vi "Test Deserialize Variant Attributes.vi"(8 "error in (no error)":errorcluster) -> (0 "error out":errorcluster)   [LabVIEW 2015]
uses:
  src/Deserializer/JSON Deserializer/JSON Deserializer.lvclass
  <vilib>/addons/_JKI Toolkits/Caraya/classes/Test/Test.lvclass
  <vilib>/addons/_JKI Toolkits/Caraya/classes/Assert/Assert.lvclass
  <vilib>/Utility/Data Type/NI_Data Type.lvlib
panel:
  out "element":variant
  out "value 2":variant
  out "data 2":string
  out "value":variant
  in  "Google reverse-geocode results":string="{\n   \"results\" : [\n      {\n         \"address_components\" : [\n            {\n               \"long_name\" : \"The White House\",\n               \"short_name\" : \"The White House\",\n               \"types\" : [ \"premise\" ]\n            },\n            {\n               \"long_name\" : \"1600\",\n               \"short_name\" : \"1600\",\n               \"types\" : [ \"street_number\" ]\n            },\n            {\n               \"long_name\" : \"Pennsylvania Avenue Northwest\",\n               \"short_name\" : \"Pennsylvania Ave NW\",\n               \"types\" : [ \"route\" ]\n            },\n            {\n               \"long_name\" : \"Northwest Washington\",\n               \"short_name\" : \"Northwest Washington\",\n               \"types\" : [ \"neighborhood\", \"political\" ]\n            },\n            {\n               \"long_name\" : \"Washington\",\n               \"short_name\" : \"Washington\",\n               \"types\" : [ \"locality\", \"political\" ]\n            },\n            {\n               \"long_name\" : \"District of Columbia\",\n               \"short_name\" : \"DC\",\n               \"types\" : [ \"administrative_area_level_1\", \"political\" ]\n            },\n            {\n               \"long_name\" : \"United States\",\n               \"short_name\" : \"US\",\n               \"types\" : [ \"country\", \"political\" ]\n            },\n            {\n               \"long_name\" : \"20500\",\n               \"short_name\" : \"20500\",\n               \"types\" : [ \"postal_code\" ]\n            }\n         ],\n         \"formatted_address\" : \"The White House, 1600 Pennsylvania Ave NW, Washington, DC 20500, USA\",\n         \"geometry\" : {\n            \"bounds\" : {\n               \"northeast\" : {\n                  \"lat\" : 38.8979044,\n                  \"lng\" : -77.0355124\n               },\n               \"southwest\" : {\n                  \"lat\" : 38.8973144,\n                  \"lng\" : -77.03795749999999\n               }\n            },\n            \"location\" : {\n               \"lat\" : 38.8976094,\n               \"lng\" : -77.0367349\n            },\n            \"location_type\" : \"ROOFTOP\",\n            \"viewport\" : {\n               \"northeast\" : {\n                  \"lat\" : 38.8989583802915,\n                  \"lng\" : -77.03538596970849\n               },\n               \"southwest\" : {\n                  \"lat\" : 38.8962604197085,\n                  \"lng\" : -77.03808393029151\n               }\n            }\n         },\n         \"place_id\" : \"ChIJGVtI4by3t4kRr51d_Qm_x58\",\n         \"types\" : [ \"premise\" ]\n      },\n      {\n         \"address_components\" : [\n            {\n               \"long_name\" : \"West Executive Avenue Northwest\",\n               \"short_name\" : \"W Executive Ave NW\",\n               \"types\" : [ \"route\" ]\n            },\n            {\n               \"long_name\" : \"Northwest Washington\",\n               \"short_name\" : \"Northwest Washington\",\n               \"types\" : [ \"neighborhood\", \"political\" ]\n            },\n            {\n               \"long_name\" : \"Washington\",\n               \"short_name\" : \"Washington\",\n               \"types\" : [ \"locality\", \"political\" ]\n            },\n            {\n               \"long_name\" : \"District of Columbia\",\n               \"short_name\" : \"DC\",\n               \"types\" : [ \"administrative_area_level_1\", \"political\" ]\n            },\n            {\n               \"long_name\" : \"United States\",\n               \"short_name\" : \"US\",\n               \"types\" : [ \"country\", \"political\" ]\n            },\n            {\n               \"long_name\" : \"20500\",\n               \"short_name\" : \"20500\",\n               \"types\" : [ \"postal_code\" ]\n            }\n         ],\n         \"formatted_address\" : \"W Executive Ave NW, Washington, DC 20500, USA\",\n         \"geometry\" : {\n            \"bounds\" : {\n               \"northeast\" : {\n                  \"lat\" : 38.8987179,\n                  \"lng\" : -77.0379902\n               },\n               \"southwest\" : {\n                  \"lat\" : 38.8963906,\n                  \"lng\" : -77.0379916\n               }\n            },\n            \"location\" : {\n               \"lat\" : 38.89755419999999,\n               \"lng\" : -77.0379909\n            },\n            \"location_type\" : \"GEOMETRIC_CENTER\",\n            \"viewport\" : {\n               \"northeast\" : {\n                  \"lat\" : 38.8989032302915,\n                  \"lng\" : -77.03664191970849\n               },\n               \"southwest\" : {\n                  \"lat\" : 38.8962052697085,\n                  \"lng\" : -77.03933988029149\n               }\n            }\n         },\n         \"place_id\" : \"ChIJPWmSlby3t4kRBbzLK31n4RE\",\n         \"types\" : [ \"route\" ]\n      },\n      {\n         \"address_components\" : [\n            {\n               \"long_name\" : \"Northwest Washington\",\n               \"short_name\" : \"Northwest Washington\",\n               \"types\" : [ \"neighborhood\", \"political\" ]\n            },\n            {\n               \"long_name\" : \"Washington\",\n               \"short_name\" : \"Washington\",\n               \"types\" : [ \"locality\", \"political\" ]\n            },\n            {\n               \"long_name\" : \"District of Columbia\",\n               \"short_name\" : \"DC\",\n               \"types\" : [ \"administrative_area_level_1\", \"political\" ]\n            },\n            {\n               \"long_name\" : \"United States\",\n               \"short_name\" : \"US\",\n               \"types\" : [ \"country\", \"political\" ]\n            }\n         ],\n         \"formatted_address\" : \"Northwest Washington, Washington, DC, USA\",\n         \"geometry\" : {\n            \"bounds\" : {\n               \"northeast\" : {\n                  \"lat\" : 38.9955566,\n                  \"lng\" : -77.00605969999999\n               },\n               \"southwest\" : {\n                  \"lat\" : 38.8891955,\n                  \"lng\" : -77.1197502\n               }\n            },\n            \"location\" : {\n               \"lat\" : 38.9380912,\n               \"lng\" : -77.04493269999999\n            },\n            \"location_type\" : \"APPROXIMATE\",\n            \"viewport\" : {\n               \"northeast\" : {\n                  \"lat\" : 38.9955566,\n                  \"lng\" : -77.00605969999999\n               },\n               \"southwest\" : {\n                  \"lat\" : 38.8891955,\n                  \"lng\" : -77.1197502\n               }\n            }\n         },\n         \"place_id\" : \"ChIJi7U4CaS3t4kR0m_KoPJ00Bw\",\n         \"types\" : [ \"neighborhood\", \"political\" ]\n      },\n      {\n         \"address_components\" : [\n            {\n               \"long_name\" : \"Washington\",\n               \"short_name\" : \"Washington\",\n               \"types\" : [ \"locality\", \"political\" ]\n            },\n            {\n               \"long_name\" : \"District of Columbia\",\n               \"short_name\" : \"District of Columbia\",\n               \"types\" : [ \"administrative_area_level_2\", \"political\" ]\n            },\n            {\n               \"long_name\" : \"District of Columbia\",\n               \"short_name\" : \"DC\",\n               \"types\" : [ \"administrative_area_level_1\", \"political\" ]\n            },\n            {\n               \"long_name\" : \"United States\",\n               \"short_name\" : \"US\",\n               \"types\" : [ \"country\", \"political\" ]\n            }\n         ],\n         \"formatted_address\" : \"Washington, DC, USA\",\n         \"geometry\" : {\n            \"bounds\" : {\n               \"northeast\" : {\n                  \"lat\" : 38.995548,\n                  \"lng\" : -76.90939299999999\n               },\n               \"southwest\" : {\n                  \"lat\" : 38.8031494,\n                  \"lng\" : -77.1197401\n               }\n            },\n            \"location\" : {\n               \"lat\" : 38.9071923,\n               \"lng\" : -77.03687069999999\n            },\n            \"location_type\" : \"APPROXIMATE\",\n            \"viewport\" : {\n               \"northeast\" : {\n                  \"lat\" : 38.995548,\n                  \"lng\" : -76.90939299999999\n               },\n               \"southwest\" : {\n                  \"lat\" : 38.8031494,\n                  \"lng\" : -77.1197401\n               }\n            }\n         },\n         \"place_id\" : \"ChIJW-T2Wt7Gt4kRKl2I1CJFUsI\",\n         \"types\" : [ \"locality\", \"political\" ]\n      },\n      {\n         \"address_components\" : [\n            {\n               \"long_name\" : \"20502\",\n               \"short_name\" : \"20502\",\n               \"types\" : [ \"postal_code\" ]\n            },\n            {\n               \"long_name\" : \"Northwest Washington\",\n               \"short_name\" : \"Northwest Washington\",\n               \"types\" : [ \"neighborhood\", \"political\" ]\n            },\n            {\n               \"long_name\" : \"Washington\",\n               \"short_name\" : \"Washington\",\n               \"types\" : [ \"locality\", \"political\" ]\n            },\n            {\n               \"long_name\" : \"District of Columbia\",\n               \"short_name\" : \"DC\",\n               \"types\" : [ \"administrative_area_level_1\", \"political\" ]\n            },\n            {\n               \"long_name\" : \"United States\",\n               \"short_name\" : \"US\",\n               \"types\" : [ \"country\", \"political\" ]\n            }\n         ],\n         \"formatted_address\" : \"Washington, DC 20502, USA\",\n         \"geometry\" : {\n            \"bounds\" : {\n               \"northeast\" : {\n                  \"lat\" : 38.898761,\n                  \"lng\" : -77.03386789999999\n               },\n               \"southwest\" : {\n                  \"lat\" : 38.8926099,\n                  \"lng\" : -77.03848579999999\n               }\n            },\n            \"location\" : {\n               \"lat\" : 38.8967584,\n               \"lng\" : -77.03701629999999\n            },\n            \"location_type\" : \"APPROXIMATE\",\n            \"viewport\" : {\n               \"northeast\" : {\n                  \"lat\" : 38.898761,\n                  \"lng\" : -77.03386789999999\n               },\n               \"southwest\" : {\n                  \"lat\" : 38.8926099,\n                  \"lng\" : -77.03848579999999\n               }\n            }\n         },\n         \"place_id\" : \"ChIJFfZlI6O3t4kRT21JVHxrwx4\",\n         \"types\" : [ \"postal_code\" ]\n      },\n      {\n         \"address_components\" : [\n            {\n               \"long_name\" : \"20372\",\n               \"short_name\" : \"20372\",\n               \"types\" : [ \"postal_code\" ]\n            },\n            {\n               \"long_name\" : \"Washington\",\n               \"short_name\" : \"Washington\",\n               \"types\" : [ \"locality\", \"political\" ]\n            },\n            {\n               \"long_name\" : \"District of Columbia\",\n               \"short_name\" : \"DC\",\n               \"types\" : [ \"administrative_area_level_1\", \"political\" ]\n            },\n            {\n               \"long_name\" : \"United States\",\n               \"short_name\" : \"US\",\n               \"types\" : [ \"country\", \"political\" ]\n            }\n         ],\n         \"formatted_address\" : \"Washington, DC 20372, USA\",\n         \"geometry\" : {\n            \"bounds\" : {\n               \"northeast\" : {\n                  \"lat\" : 38.9103761,\n                  \"lng\" : -77.00899819999999\n               },\n               \"southwest\" : {\n                  \"lat\" : 38.8822807,\n                  \"lng\" : -77.0576224\n               }\n            },\n            \"location\" : {\n               \"lat\" : 38.8992416,\n               \"lng\" : -77.0303423\n            },\n            \"location_type\" : \"APPROXIMATE\",\n            \"viewport\" : {\n               \"northeast\" : {\n                  \"lat\" : 38.9103761,\n                  \"lng\" : -77.00899819999999\n               },\n               \"southwest\" : {\n                  \"lat\" : 38.8822807,\n                  \"lng\" : -77.0576224\n               }\n            }\n         },\n         \"place_id\" : \"ChIJGzCb9gq4t4kRN_0lpRhRhjU\",\n         \"types\" : [ \"postal_code\" ]\n      },\n      {\n         \"address_components\" : [\n            {\n               \"long_name\" : \"District of Columbia\",\n               \"short_name\" : \"DC\",\n               \"types\" : [ \"administrative_area_level_1\", \"political\" ]\n            },\n            {\n               \"long_name\" : \"United States\",\n               \"short_name\" : \"US\",\n               \"types\" : [ \"country\", \"political\" ]\n            }\n         ],\n         \"formatted_address\" : \"District of Columbia, USA\",\n         \"geometry\" : {\n            \"bounds\" : {\n               \"northeast\" : {\n                  \"lat\" : 38.995548,\n                  \"lng\" : -76.90939299999999\n               },\n               \"southwest\" : {\n                  \"lat\" : 38.8031494,\n                  \"lng\" : -77.1197401\n               }\n            },\n            \"location\" : {\n               \"lat\" : 38.9059849,\n               \"lng\" : -77.03341790000002\n            },\n            \"location_type\" : \"APPROXIMATE\",\n            \"viewport\" : {\n               \"northeast\" : {\n                  \"lat\" : 38.995548,\n                  \"lng\" : -76.90939299999999\n               },\n               \"southwest\" : {\n                  \"lat\" : 38.8031494,\n                  \"lng\" : -77.1197401\n               }\n            }\n         },\n         \"place_id\" : \"ChIJW-T2Wt7Gt4kRmKFUAsCO4tY\",\n         \"types\" : [ \"administrative_area_level_1\", \"political\" ]\n      },\n      {\n         \"address_components\" : [\n            {\n               \"long_name\" : \"Washington-Arlington-Alexandria, DC-VA-MD-WV\",\n               \"short_name\" : \"Washington-Arlington-Alexandria, DC-VA-MD-WV\",\n               \"types\" : [ \"political\" ]\n            },\n            {\n               \"long_name\" : \"United States\",\n               \"short_name\" : \"US\",\n               \"types\" : [ \"country\", \"political\" ]\n            }\n         ],\n         \"formatted_address\" : \"Washington-Arlington-Alexandria, DC-VA-MD-WV, USA\",\n         \"geometry\" : {\n            \"bounds\" : {\n               \"northeast\" : {\n                  \"lat\" : 39.720018,\n                  \"lng\" : -76.38622889999999\n               },\n               \"southwest\" : {\n                  \"lat\" : 37.9911599,\n                  \"lng\" : -78.38668199999999\n               }\n            },\n            \"location\" : {\n               \"lat\" : 39.1289725,\n               \"lng\" : -77.3783789\n            },\n            \"location_type\" : \"APPROXIMATE\",\n            \"viewport\" : {\n               \"northeast\" : {\n                  \"lat\" : 39.720023,\n                  \"lng\" : -76.38622889999999\n               },\n               \"southwest\" : {\n                  \"lat\" : 37.9911599,\n                  \"lng\" : -78.38668199999999\n               }\n            }\n         },\n         \"place_id\" : \"ChIJy25QE7lFtokRgaAnbc9iMr8\",\n         \"types\" : [ \"political\" ]\n      },\n      {\n         \"address_components\" : [\n            {\n               \"long_name\" : \"United States\",\n               \"short_name\" : \"US\",\n               \"types\" : [ \"country\", \"political\" ]\n            }\n         ],\n         \"formatted_address\" : \"United States\",\n         \"geometry\" : {\n            \"bounds\" : {\n               \"northeast\" : {\n                  \"lat\" : 71.3867745,\n                  \"lng\" : -66.9502861\n               },\n               \"southwest\" : {\n                  \"lat\" : 18.910677,\n                  \"lng\" : 172.4458955\n               }\n            },\n            \"location\" : {\n               \"lat\" : 37.09024,\n               \"lng\" : -95.712891\n            },\n            \"location_type\" : \"APPROXIMATE\",\n            \"viewport\" : {\n               \"northeast\" : {\n                  \"lat\" : 49.38,\n                  \"lng\" : -66.94\n               },\n               \"southwest\" : {\n                  \"lat\" : 25.82,\n                  \"lng\" : -124.39\n               }\n            }\n         },\n         \"place_id\" : \"ChIJCzYy5IS16lQRQrfeQ5K5Oxw\",\n         \"types\" : [ \"country\", \"political\" ]\n      }\n   ],\n   \"status\" : \"OK\"\n}\n"
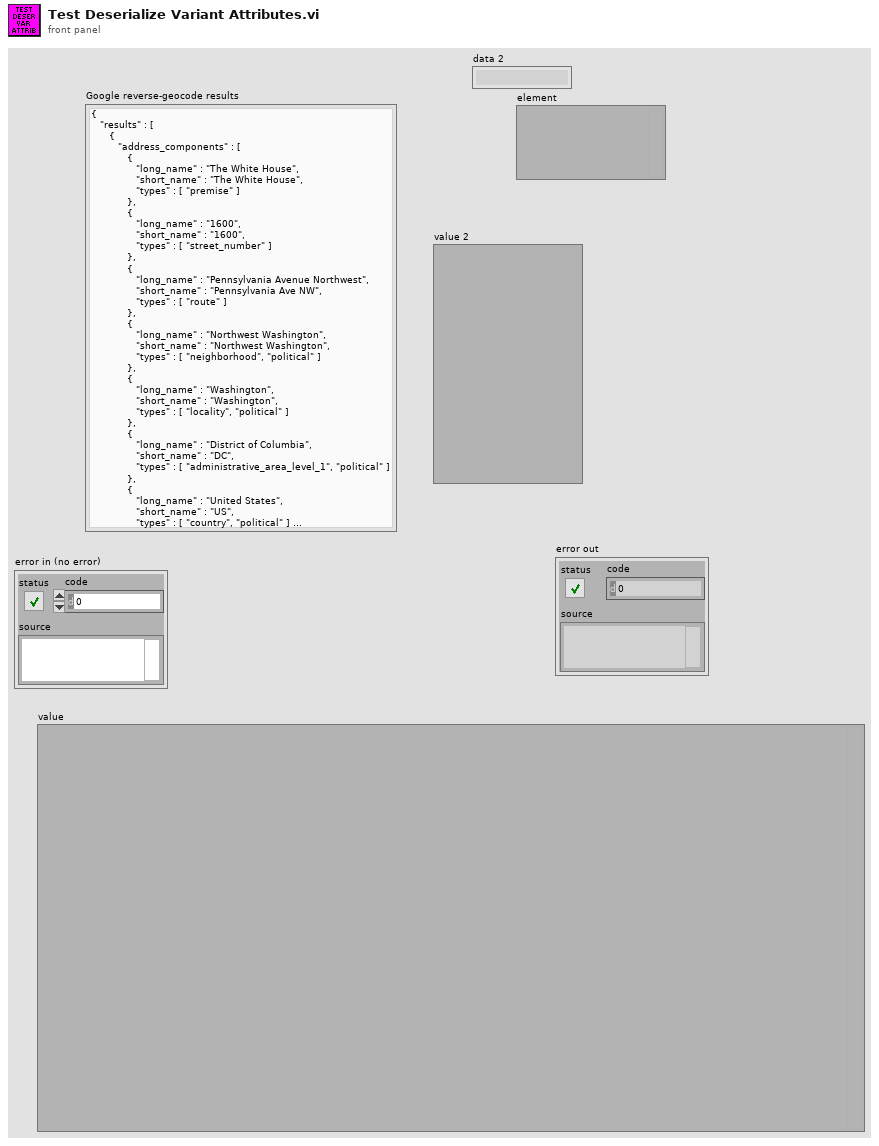
[diagram p1: front panel]
types:
  T1 = typedef "NI_Data Type.lvlib/Data Type.ctl" = enum8{"Invalid Type", "Void", "I8", "I16", "I32", "I64", "U8", "U16", "U32", "U64", "Single Float", "Double Float", "Extended Float", "Single Complex", "Double Complex", "Extended Complex", "Enum U8", "Enum U16", "Enum U32", "Enum U64", "Single Float With Unit", "Double Float With Unit", "Extended Float With Unit", "Single Complex with Unit", "Double Complex with Unit", "Extended Complex with Unit", "Boolean", "String", "Path", "Picture", "Tag", "Array", "Cluster", "Variant", "LV Variant", "Waveform", "Timestamp", "Digital Waveform", "Digital Data", "ExpressData", "Refnum", "External Data", "VI", "Poly VI", "LabVIEW Class Instance", "Fixed Point"}
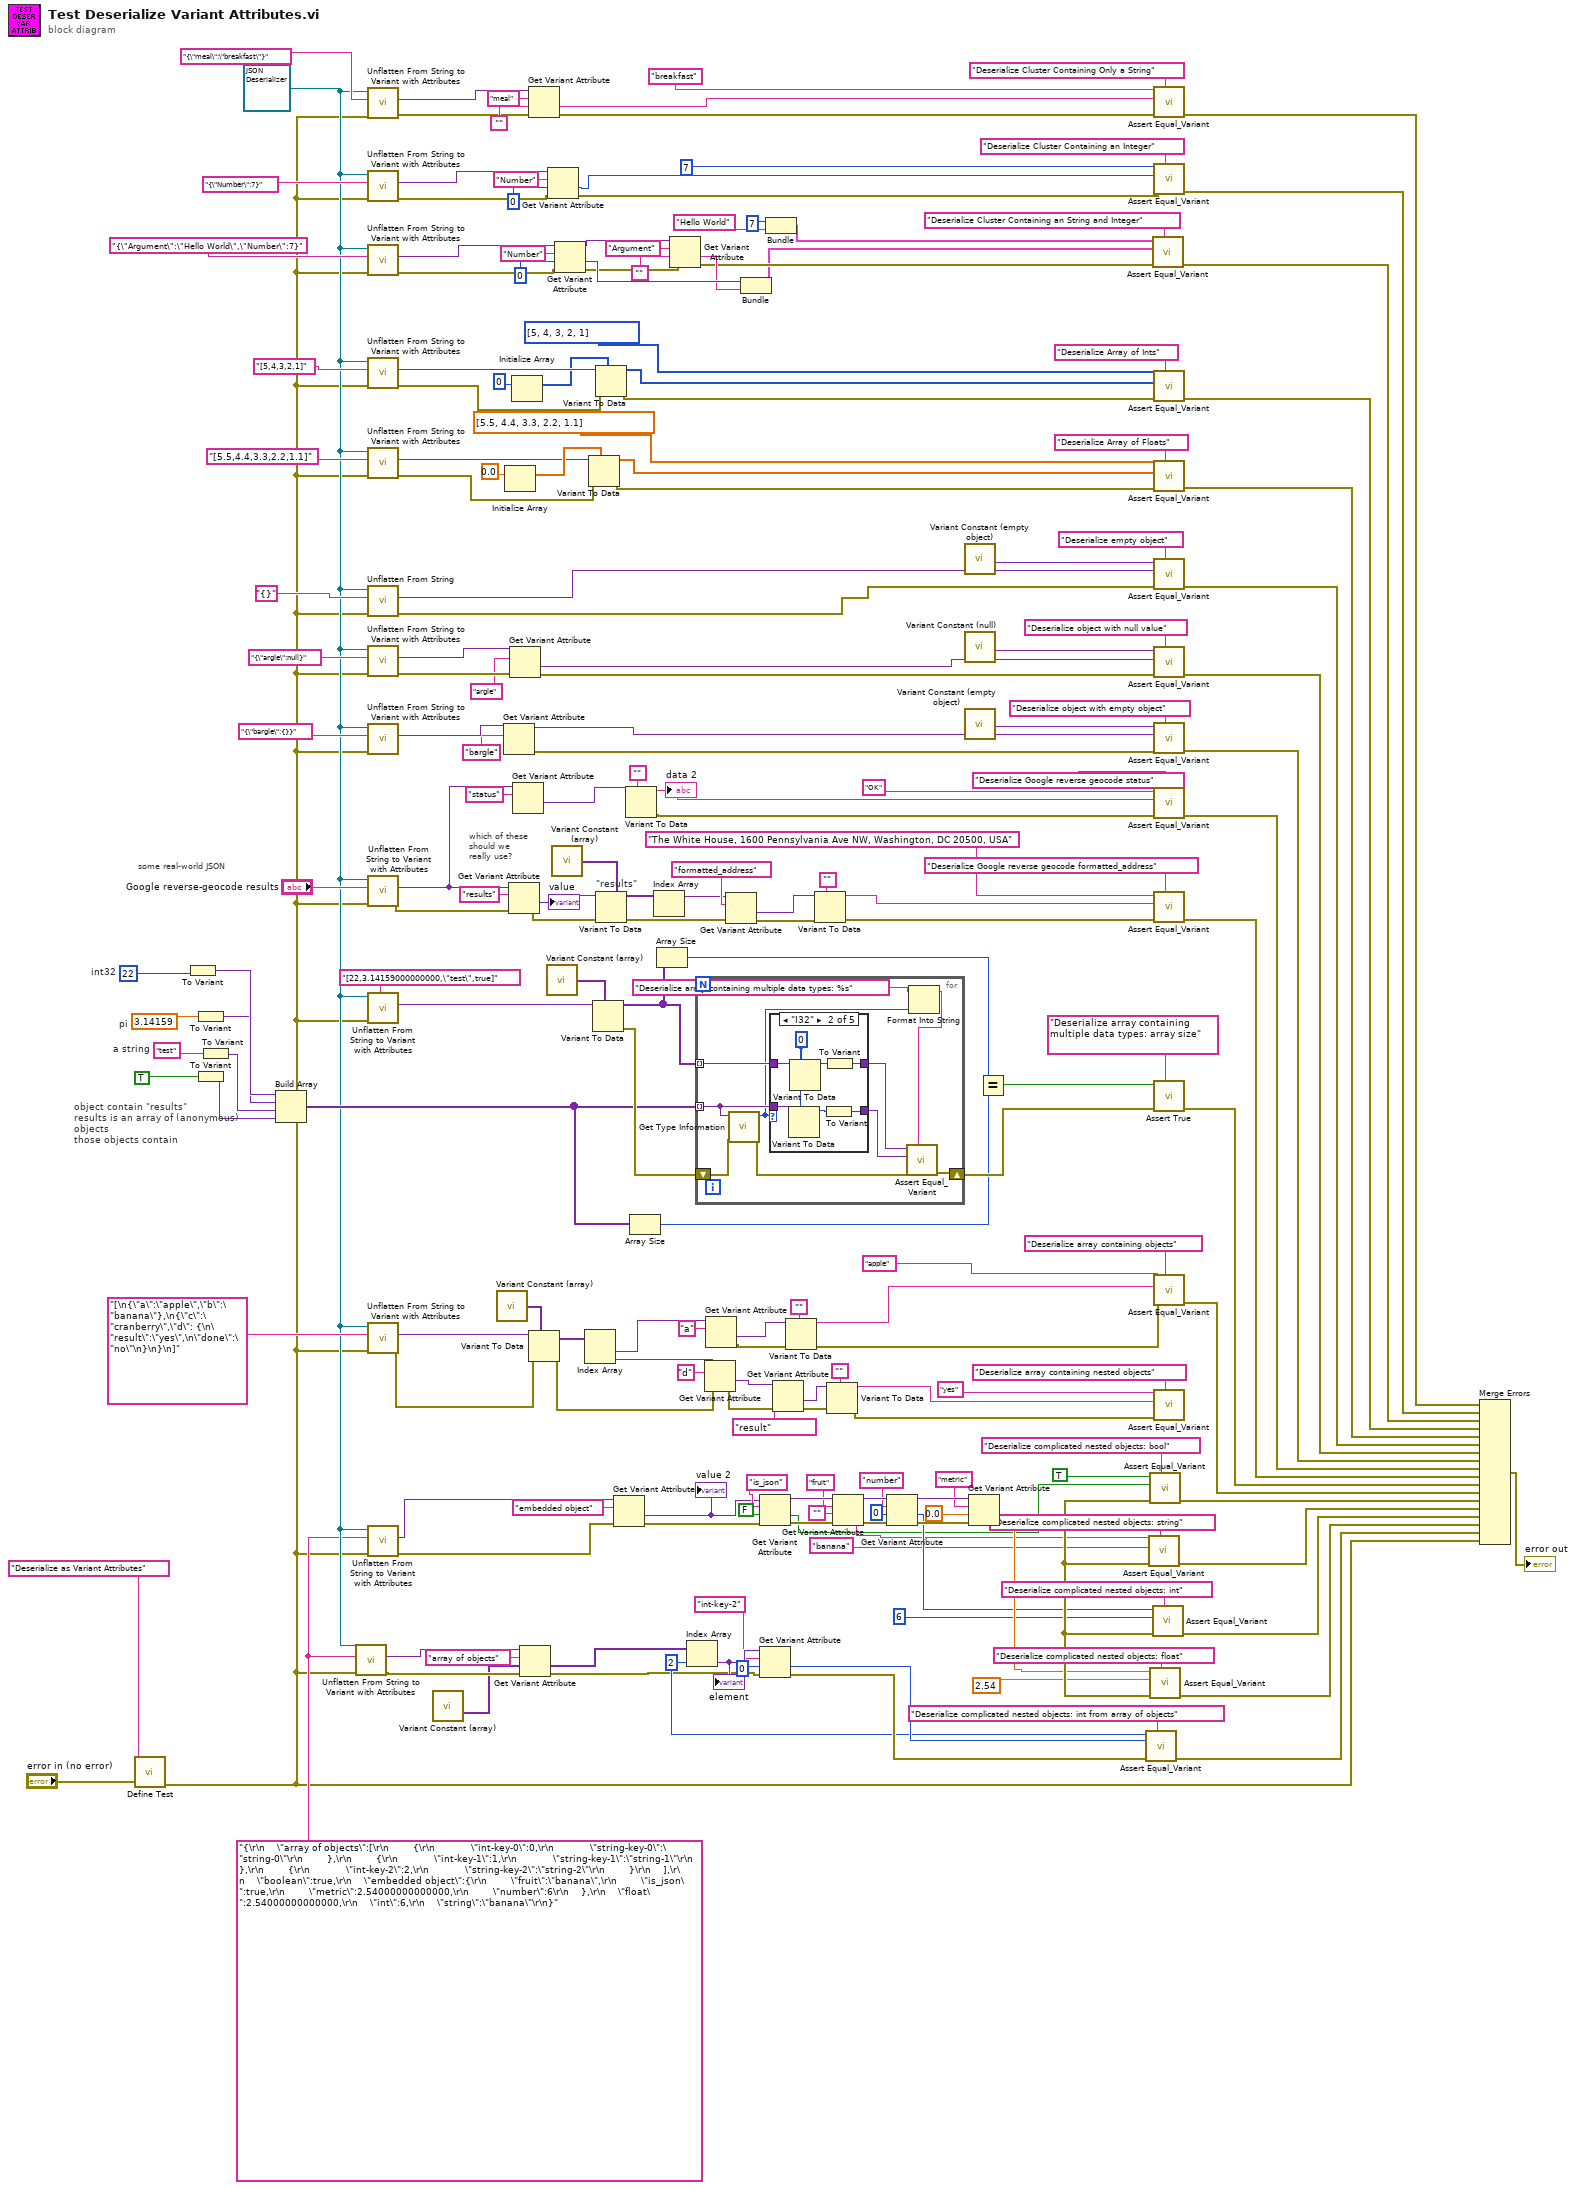
[diagram p0: block diagram]
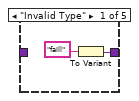
[diagram p2: hidden frame]
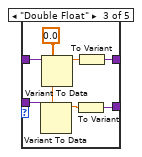
[diagram p3: hidden frame]
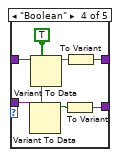
[diagram p4: hidden frame]
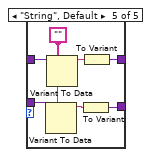
[diagram p5: hidden frame]
diagram:
  w9 = 2 ("index")
  w16 = "{\r\n    \"array of objects\":[\r\n        {\r\n            \"int-key-0\":0,\r\n            \"string-key-0\":\"string-0\"\r\n        },\r\n        {\r\n            \"int-key-1\":1,\r\n            \"string-key-1\":\"string-1\"\r\n        },\r\n        {\r\n            \"int-key-2\":2,\r\n            \"string-key-2\":\"string-2\"\r\n        }\r\n    ],\r\n    \"boolean\":true,\r\n    \"embedded object\":{\r\n        \"fruit\":\"banana\",\r\n        \"is_json\":true,\r\n        \"metric\":2.54000000000000,\r\n        \"number\":6\r\n    },\r\n    \"float\":2.54000000000000,\r\n    \"int\":6,\r\n    \"string\":\"banana\"\r\n}" ("String")
  w17 = refnum<class "JSON Deserializer.lvclass"> refnum ("Deserializer out")
  w194 = "test"  # a string
  w190 = 3.14159  # pi
  w195 = 22  # int32
  # "which of these\nshould we \nreally use?"
  # "some real-world JSON"
  # "object contain \"results\"\nresults is an array of (anonymous) objects\nthose objects contain"
  n1 = call <vilib>:"Define Test.vi"("error in (no error)"="error in (no error)", "Label (VI Title)"="Deserialize as Variant Attributes") -> ("error out"=w1:errorcluster)  [unwired: 9 in]
  n2 = To Variant(anything=w195) -> (Variant=w193:variant)
  n3 = To Variant(anything=w190) -> (Variant=w192:variant)
  n4 = To Variant(anything=TRUE) -> (Variant=w188:variant)
  n5 = To Variant(anything=w194) -> (Variant=w191:variant)
  n6 = Build Array(w193, w192, w191, w188) -> (w113:variant[])
  n7 = call-dynamic "Unflatten From String to Variant with Attributes.vi"("error in (no error)"=w1, "String"=w16, "Deserializer in"=w17) -> ("error out"=w7:errorcluster, "Variant with Attributes"=w6:variant)  [unwired: 6 in, 1 out]
  n8 = call-dynamic "Unflatten From String to Variant with Attributes.vi"("error in (no error)"=w1, "String"="{\"meal\":\"breakfast\"}" ("String 2"), "Deserializer in"=w17) -> ("error out"=w159:errorcluster, "Variant with Attributes"=w161:variant)  [unwired: 6 in, 1 out]
  n9 = call-dynamic "Unflatten From String to Variant with Attributes.vi"("error in (no error)"=w1, "String"="{\"Number\":7}", "Deserializer in"=w17) -> ("error out"=w149:errorcluster, "Variant with Attributes"=w132:variant)  [unwired: 6 in, 1 out]
  n10 = call-dynamic "Unflatten From String to Variant with Attributes.vi"("error in (no error)"=w1, "String"="{\"Argument\":\"Hello World\",\"Number\":7}", "Deserializer in"=w17) -> ("error out"=w148:errorcluster, "Variant with Attributes"=w133:variant)  [unwired: 6 in, 1 out]
  n11 = call-dynamic "Unflatten From String to Variant with Attributes.vi"("error in (no error)"=w1, "String"="[5,4,3,2,1]", "Deserializer in"=w17) -> ("error out"=w168:errorcluster, "Variant with Attributes"=w173:variant)  [unwired: 6 in, 1 out]
  n12 = call-dynamic "Unflatten From String to Variant with Attributes.vi"("error in (no error)"=w1, "String"="[5.5,4.4,3.3,2.2,1.1]", "Deserializer in"=w17) -> ("error out"=w76:errorcluster, "Variant with Attributes"=w71:variant)  [unwired: 6 in, 1 out]
  n13 = call-dynamic "Unflatten From String.vi"("error in (no error)"=w1, "String"="{}", "Deserializer in"=w17) -> ("error out"=w78:errorcluster, "Variant"=w81:variant)  [unwired: 6 in, 1 out]
  n14 = call-dynamic "Unflatten From String to Variant with Attributes.vi"("error in (no error)"=w1, "String"="{\"argle\":null}" ("JSON String 2"), "Deserializer in"=w17) -> ("error out"=w209:errorcluster, "Variant with Attributes"=w208:variant)  [unwired: 6 in, 1 out]
  n15 = call-dynamic "Unflatten From String to Variant with Attributes.vi"("error in (no error)"=w1, "String"="{\"bargle\":{}}" ("JSON String 2"), "Deserializer in"=w17) -> ("Variant with Attributes"=w202:variant)  [unwired: 6 in, 2 out]
  n16 = call-dynamic "Unflatten From String to Variant with Attributes.vi"("error in (no error)"=w1, "String"="Google reverse-geocode results", "Deserializer in"=w17) -> ("error out"=w125:errorcluster, "Variant with Attributes"=w180:variant)  [unwired: 6 in, 1 out]
  n17 = call-dynamic "Unflatten From String to Variant with Attributes.vi"("error in (no error)"=w1, "String"="[22,3.14159000000000,\"test\",true]", "Deserializer in"=w17) -> ("Variant with Attributes"=w186:variant)  [unwired: 6 in, 2 out]
  n18 = call-dynamic "Unflatten From String to Variant with Attributes.vi"("error in (no error)"=w1, "String"="[\n{\"a\":\"apple\",\"b\":\"banana\"},\n{\"c\":\"cranberry\",\"d\": {\n\"result\":\"yes\",\n\"done\":\"no\"\n}\n}\n]", "Deserializer in"=w17) -> ("error out"=w95:errorcluster, "Variant with Attributes"=w107:variant)  [unwired: 6 in, 1 out]
  n19 = call-dynamic "Unflatten From String to Variant with Attributes.vi"("error in (no error)"=w1, "String"=w16, "Deserializer in"=w17) -> ("error out"=w22:errorcluster, "Variant with Attributes"=w21:variant)  [unwired: 6 in, 1 out]
  n20 = call "Variant Constant (array).vi"() -> ("array"=w4:variant[])  [unwired: 2 in]
  n21 = call "Variant Constant (array).vi"() -> ("array"=w18:variant[])  [unwired: 2 in]
  n22 = Get Variant Attribute(Variant=w202, name="bargle") -> (duplicate Variant=w199:variant, error out=w131:errorcluster)  [unwired: 2 in, 2 out]
  n23 = Initialize Array(0.0) -> (w74:dbl[])  [unwired: 1 in]
  n24 = Get Variant Attribute(Variant=w180, name="results", error in=w125) -> (value=w184:variant, error out=w124:errorcluster)  [unwired: 1 in, 2 out]
  "value" <- w184
  n25 = Get Variant Attribute(Variant=w208, name="argle", error in=w209) -> (value=w205:variant, error out=w206:errorcluster)  [unwired: 1 in, 2 out]
  n26 = Initialize Array(0) -> (w170:i32[])  [unwired: 1 in]
  n27 = Get Variant Attribute(Variant=w180, name="status") -> (value=w178:variant)  [unwired: 2 in, 3 out]
  n28 = Get Variant Attribute(Variant=w6, name="array of objects", default value (empty Variant)=w4, error in=w7) -> (value=w2:variant[], error out=w3:errorcluster)  [unwired: 2 out]
  n29 = Get Variant Attribute(Variant=w161, name="meal", default value (empty Variant)="", error in=w159) -> (value=w157:string, error out=w158:errorcluster)  [unwired: 2 out]
  n30 = Variant To Data(error in=w95, type=w18, Variant=w107) -> (data=w106:variant[], error out=w96:errorcluster)
  n31 = call "Variant Constant (array).vi"() -> ("array"=w20:variant[])  [unwired: 2 in]
  n32 = Get Variant Attribute(Variant=w132, name="Number", default value (empty Variant)=0, error in=w149) -> (value=w151:i32, error out=w150:errorcluster)  [unwired: 2 out]
  n33 = call "Variant Constant (array).vi"() -> ("array"=w19:variant[])  [unwired: 2 in]
  n34 = Get Variant Attribute(Variant=w133, name="Number", default value (empty Variant)=0, error in=w148) -> (duplicate Variant=w143:variant, value=w141:i32, error out=w137:errorcluster)  [unwired: 1 out]
  n35 = Index Array(array=w106) -> (element #1=w93:variant, element #2=w108:variant)  [unwired: 2 in]
  n36 = Variant To Data(error in=w76, type=w74, Variant=w71) -> (data=w75:dbl[], error out=w77:errorcluster)
  n37 = Variant To Data(type=w20, Variant=w186) -> (data=w117:variant[], error out=w115:errorcluster)  [unwired: 1 in]
  n38 = Variant To Data(error in=w168, type=w170, Variant=w173) -> (data=w169:i32[], error out=w167:errorcluster)
  n39 = Variant To Data "\"results\""(error in=w124, type=w19, Variant=w184) -> (data=w183:variant[], error out=w123:errorcluster)
  n40 = Get Variant Attribute(Variant=w21, name="embedded object", error in=w22) -> (value=w44:variant, error out=w43:errorcluster)  [unwired: 1 in, 2 out]
  "value 2" <- w44
  n41 = Variant To Data(type="", Variant=w178) -> (data=w129:string, error out=w130:errorcluster)  [unwired: 1 in]
  "data 2" <- w129
  n42 = Array Size(array=w113) -> (size(s)=w112:i32)
  n43 = Index Array(array=w183) -> (element=w176:variant)  [unwired: 1 in]
  n44 = Array Size(array=w117) -> (size(s)=w116:i32)
  n45 = Get Variant Attribute(Variant=w143, name="Argument", default value (empty Variant)="", error in=w137) -> (value=w140:string, error out=w136:errorcluster)  [unwired: 2 out]
  n46 = Index Array(array=w2, index=w9) -> (element=w15:variant)
  "element" <- w15
  n47 = for {
    tunnel: w113 -> [w221] mode=indexing
    tunnel: w117 -> [w222] mode=indexing
    shift-right: [w218] -> w114
    shift-left: w115 -> [w220]
    n48 = call <vilib>:"Get Type Information.vi"("error in (no error)"=w220, "Variant"=w221) -> ("error out"=w219:errorcluster, "Type"=w214:T1)  [unwired: 5 in, 3 out]
    n49 = case shown="\"I32\"" w214 {
      tunnel: w222 -> [_ w231 w238 w245 w252]
      tunnel: w221 -> [_ w230 w237 w244 w251]
      tunnel: [w223 w228 w235 w242 w249] -> w217
      tunnel: [_ w226 w233 w240 w247] -> w216
      frame "Invalid Type" {
        n50 = To Variant(anything="faill" ("name")) -> (Variant=w223:variant)
      }
      frame "I32" {
        w225 = 0
        n51 = Variant To Data(type=w225, Variant=w230) -> (data=w227:i32)  [unwired: 1 in, 1 out]
        n52 = Variant To Data(type=w225, Variant=w231) -> (data=w229:i32)  [unwired: 1 in, 1 out]
        n53 = To Variant(anything=w227) -> (Variant=w226:variant)
        n54 = To Variant(anything=w229) -> (Variant=w228:variant)
      }
      frame "Double Float" {
        w232 = 0.0
        n55 = Variant To Data(type=w232, Variant=w237) -> (data=w234:dbl)  [unwired: 1 in, 1 out]
        n56 = Variant To Data(type=w232, Variant=w238) -> (data=w236:dbl)  [unwired: 1 in, 1 out]
        n57 = To Variant(anything=w234) -> (Variant=w233:variant)
        n58 = To Variant(anything=w236) -> (Variant=w235:variant)
      }
      frame "Boolean" {
        w239 = TRUE
        n59 = Variant To Data(type=w239, Variant=w244) -> (data=w241:bool)  [unwired: 1 in, 1 out]
        n60 = Variant To Data(type=w239, Variant=w245) -> (data=w243:bool)  [unwired: 1 in, 1 out]
        n61 = To Variant(anything=w241) -> (Variant=w240:variant)
        n62 = To Variant(anything=w243) -> (Variant=w242:variant)
      }
      frame "String", Default {
        w246 = ""
        n63 = Variant To Data(type=w246, Variant=w251) -> (data=w248:string)  [unwired: 1 in, 1 out]
        n64 = Variant To Data(type=w246, Variant=w252) -> (data=w250:string)  [unwired: 1 in, 1 out]
        n65 = To Variant(anything=w248) -> (Variant=w247:variant)
        n66 = To Variant(anything=w250) -> (Variant=w249:variant)
      }
    }
    n67 = Format Into String(format string="Deserialize array containing multiple data types: %s" ("Label"), w214) -> (resulting string=w213:string)  [unwired: 2 in, 1 out]
    n68 = call <vilib>:"Assert Equal_Variant.vi"("Label"=w213, "error in (no error)"=w219, "Y"=w216, "X"=w217) -> ("error out"=w218:errorcluster)  [unwired: 7 in]
  }
  n69 = Get Variant Attribute(Variant=w108, name="d", error in=w96) -> (value=w110:variant, error out=w97:errorcluster)  [unwired: 1 in, 2 out]
  n70 = Get Variant Attribute(Variant=w93, name="a") -> (value=w90:variant, error out=w91:errorcluster)  [unwired: 2 in, 2 out]
  n71 = Get Variant Attribute(Variant=w176, name="formatted_address", error in=w123) -> (value=w177:variant, error out=w122:errorcluster)  [unwired: 1 in, 2 out]
  n72 = Bundle(w141, w140) -> (w134:cluster{i32, string})  [unwired: 1 in]
  n73 = Get Variant Attribute(Variant=w44, name="is_json", default value (empty Variant)=FALSE, error in=w43) -> (duplicate Variant=w52:variant, value=w23:bool, error out=w45:errorcluster)  [unwired: 1 out]
  n74 = Get Variant Attribute(Variant=w15, name="int-key-2", default value (empty Variant)=0 ("index"), error in=w3) -> (value=w10:i32, error out=w12:errorcluster)  [unwired: 2 out]
  n75 = Bundle(7, "name"="Hello World") -> (w135:cluster{i32, "name":string})  [unwired: 1 in]
  n76 = Get Variant Attribute(Variant=w110, name="result", error in=w97) -> (value=w102:variant, error out=w103:errorcluster)  [unwired: 1 in, 2 out]
  n77 = Variant To Data(error in=w91, type="", Variant=w90) -> (data=w88:string, error out=w87:errorcluster)
  n78 = Variant To Data(error in=w122, type="", Variant=w177) -> (data=w126:string, error out=w121:errorcluster)
  n79 = Variant To Data(error in=w103, type="", Variant=w102) -> (data=w100:string, error out=w98:errorcluster)
  n80 = Get Variant Attribute(Variant=w52, name="fruit", default value (empty Variant)="", error in=w45) -> (duplicate Variant=w53:variant, value=w25:string, error out=w46:errorcluster)  [unwired: 1 out]
  n81 = Get Variant Attribute(Variant=w53, name="number", default value (empty Variant)=0, error in=w46) -> (duplicate Variant=w54:variant, value=w27:i32, error out=w47:errorcluster)  [unwired: 1 out]
  n82 = call "Variant Constant (empty object).vi"() -> ("Empty Object"=w80:variant)  [unwired: 2 in]
  n83 = call "Variant Constant (null).vi"() -> ("null"=w83:variant)  [unwired: 2 in]
  n84 = call "Variant Constant (empty object).vi"() -> ("Empty Object"=w85:variant)  [unwired: 2 in]
  n85 = Get Variant Attribute(Variant=w54, name="metric", default value (empty Variant)=0.0, error in=w47) -> (value=w29:dbl, error out=w31:errorcluster)  [unwired: 2 out]
  n86 = Equal?(x=w116, y=w112) -> (x = y?=w185:bool)
  n87 = call <vilib>:"Assert Equal_Variant.vi"("Label"="Deserialize complicated nested objects: int from array of objects", "error in (no error)"=w12, "Y"=w10, "X"=w9) -> ("error out"=w11:errorcluster)  [unwired: 7 in]
  n88 = call <vilib>:"Assert Equal_Variant.vi"("Label"="Deserialize complicated nested objects: string", "error in (no error)"=w31, "Y"="banana" ("name"), "X"=w25) -> ("error out"=w37:errorcluster)  [unwired: 7 in]
  n89 = call <vilib>:"Assert Equal_Variant.vi"("Label"="Deserialize complicated nested objects: bool", "error in (no error)"=w31, "Y"=w23, "X"=TRUE) -> ("error out"=w56:errorcluster)  [unwired: 7 in]
  n90 = call <vilib>:"Assert Equal_Variant.vi"("Label"="Deserialize complicated nested objects: float", "error in (no error)"=w31, "Y"=2.54, "X"=w29) -> ("error out"=w35:errorcluster)  [unwired: 7 in]
  n91 = call <vilib>:"Assert Equal_Variant.vi"("Label"="Deserialize Cluster Containing an String and Integer", "error in (no error)"=w136, "Y"=w134, "X"=w135) -> ("error out"=w66:errorcluster)  [unwired: 7 in]
  n92 = call <vilib>:"Assert Equal_Variant.vi"("Label"="Deserialize complicated nested objects: int", "error in (no error)"=w31, "Y"=6, "X"=w27) -> ("error out"=w36:errorcluster)  [unwired: 7 in]
  n93 = call <vilib>:"Assert Equal_Variant.vi"("Label"="Deserialize Cluster Containing Only a String", "error in (no error)"=w158, "Y"=w157, "X"="breakfast" ("name")) -> ("error out"=w68:errorcluster)  [unwired: 7 in]
  n94 = call <vilib>:"Assert Equal_Variant.vi"("Label"="Deserialize Cluster Containing an Integer", "error in (no error)"=w150, "Y"=w151, "X"=7) -> ("error out"=w67:errorcluster)  [unwired: 7 in]
  n95 = call <vilib>:"Assert Equal_Variant.vi"("Label"="Deserialize Array of Ints", "error in (no error)"=w167, "Y"=w169, "X"=i32[] [5, 4, 3, 2, 1]) -> ("error out"=w65:errorcluster)  [unwired: 7 in]
  n96 = call <vilib>:"Assert Equal_Variant.vi"("Label"="Deserialize Array of Floats", "error in (no error)"=w77, "Y"=w75, "X"=dbl[] [5.5, 4.4, 3.3, 2.2, 1.1]) -> ("error out"=w64:errorcluster)  [unwired: 7 in]
  n97 = call <vilib>:"Assert Equal_Variant.vi"("Label"="Deserialize empty object" ("name"), "error in (no error)"=w78, "Y"=w81, "X"=w80) -> ("error out"=w63:errorcluster)  [unwired: 7 in]
  n98 = call <vilib>:"Assert Equal_Variant.vi"("Label"="Deserialize object with null value", "error in (no error)"=w206, "Y"=w205, "X"=w83) -> ("error out"=w62:errorcluster)  [unwired: 7 in]
  n99 = call <vilib>:"Assert Equal_Variant.vi"("Label"="Deserialize object with empty object", "error in (no error)"=w131, "Y"=w199, "X"=w85) -> ("error out"=w61:errorcluster)  [unwired: 7 in]
  n100 = call <vilib>:"Assert Equal_Variant.vi"("Label"="Deserialize Google reverse geocode status", "error in (no error)"=w130, "Y"=w129, "X"="OK" ("data 3")) -> ("error out"=w60:errorcluster)  [unwired: 7 in]
  n101 = call <vilib>:"Assert Equal_Variant.vi"("Label"="Deserialize Google reverse geocode formatted_address", "error in (no error)"=w121, "Y"=w126, "X"="The White House, 1600 Pennsylvania Ave NW, Washington, DC 20500, USA" ("data 3")) -> ("error out"=w59:errorcluster)  [unwired: 7 in]
  n102 = call <vilib>:"Assert True.vi"("Label"="Deserialize array containing multiple data types: array size", "error in (no error)"=w114, "True?"=w185) -> ("error out"=w58:errorcluster)  [unwired: 8 in]
  n103 = call <vilib>:"Assert Equal_Variant.vi"("Label"="Deserialize array containing objects", "error in (no error)"=w87, "Y"=w88, "X"="apple" ("name")) -> ("error out"=w57:errorcluster)  [unwired: 7 in]
  n104 = call <vilib>:"Assert Equal_Variant.vi"("Label"="Deserialize array containing nested objects", "error in (no error)"=w98, "Y"=w100, "X"="yes" ("name")) -> ()  [unwired: 7 in, 1 out]
  n105 = Merge Errors(w68, w67, w66, w65, w64, w63, w62, w61, w60, w59, w58, w57, w56, w37, w36, w35, w11, w1) -> (→"error out":errorcluster)
